vi "Points to Line Equation.vi"(10 "Point 2":cluster{"Global X":dbl, "Global Y":dbl}, 11 "Point 1":cluster{"Global X":dbl, "Global Y":dbl}) -> (3 "Line Equation":cluster{"m":dbl, "c":dbl})   [LabVIEW 2012]
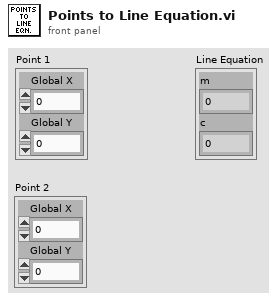
[diagram p1: front panel]
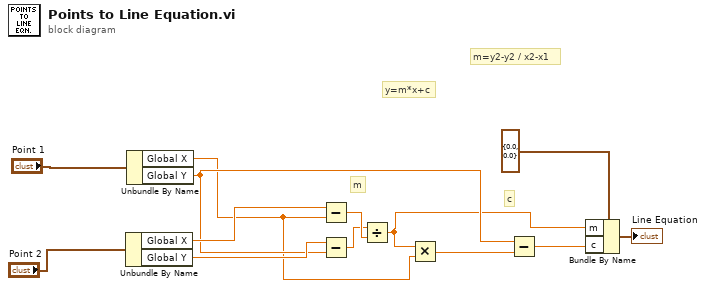
[diagram p0: block diagram]
diagram:
  # "c"
  # "m"
  # "m=y2-y2 / x2-x1"
  # "y=m*x+c"
  n1 = Unbundle By Name("Point 2") -> ("Global X"=w11:dbl, "Global Y"=w10:dbl)
  n2 = Unbundle By Name("Point 1") -> ("Global X"=w8:dbl, "Global Y"=w9:dbl)
  n3 = Subtract(x=w11, y=w8) -> (x-y=w2:dbl)
  n4 = Subtract(x=w10, y=w9) -> (x-y=w1:dbl)
  n5 = Divide(x=w1, y=w2) -> (x/y=w6:dbl)
  n6 = Multiply(x=w6, y=w8) -> (x*y=w7:dbl)
  n7 = Subtract(x=w9, y=w7) -> (x-y=w5:dbl)
  n8 = Bundle By Name(cluster=cluster{"m":dbl, "c":dbl} {"m"=0.0, "c"=0.0} ("input cluster"), "m"=w6, "c"=w5) -> (→"Line Equation":cluster{"m":dbl, "c":dbl})
